vi "Tosca-2P-Globals.vi"() -> ()   [LabVIEW 2020]
panel:
  out "Offset (s)":dbl
  out "Frame Rate (Hz)":dbl=nan
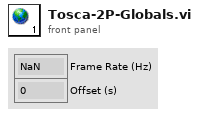
[diagram p1: front panel]
diagram:
